vi "子VI-读取缺陷测量长宽和面积.vi"(10 "Particle Reports (Pixels)":T1(array[cluster]) {"Orientation" format="%.2f"; "Dimensions"."Height" format="%.2f"; "Dimensions"."Width" format="%.2f"; "Center of Mass"."Y" format="%.2f"; "Center of Mass"."X" format="%.2f"; "Bounding Rect"."Bottom" format="%.2f"; "Bounding Rect"."Right" format="%.2f"; "Bounding Rect"."Top" format="%.2f"; "Bounding Rect"."Left" format="%.2f"; "Number of Holes" format="%.2f"; "Area" format="%.2f"}) -> (2 "测量结果":dbl[][](array[numeric]))   [LabVIEW 2018]
panel:
  out "补几列空数字":dbl[](array[numeric])
  out "高":dbl[](array[numeric])
  out "宽":dbl[](array[numeric])
  out "面积":dbl[](array[numeric])
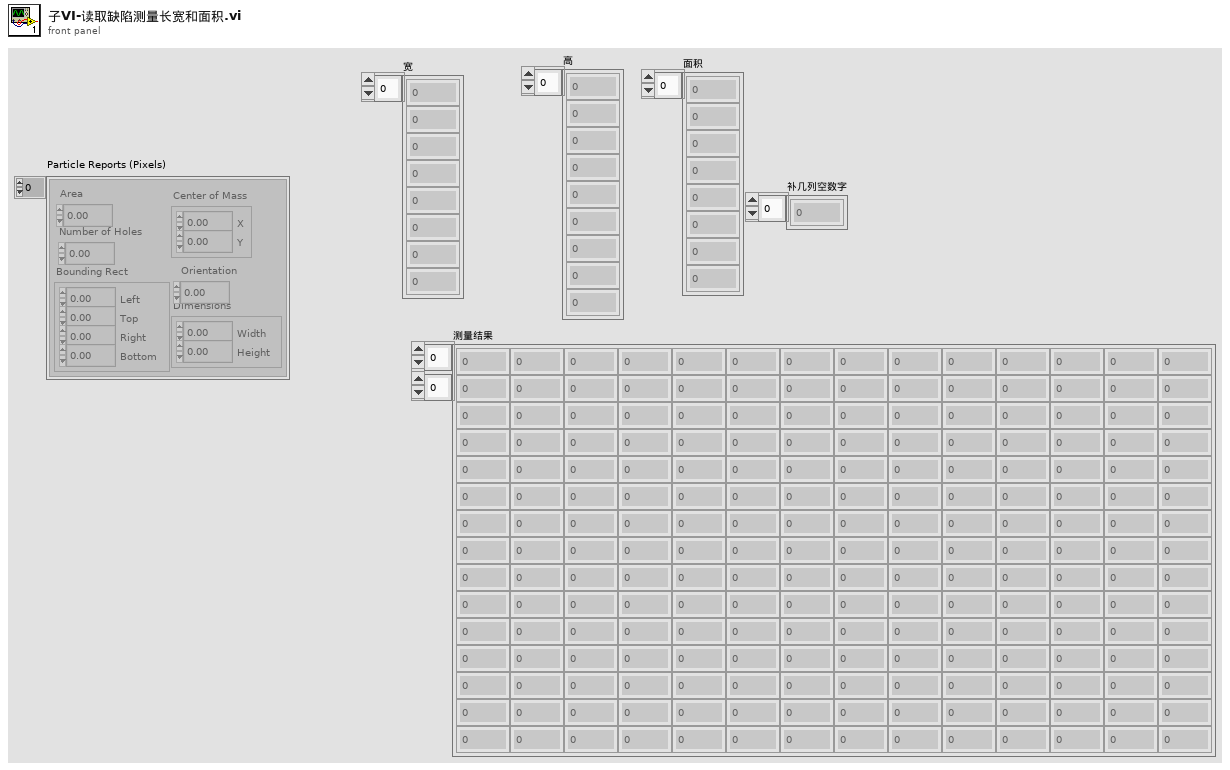
[diagram p1: front panel]
types:
  T1 = cluster{"Area":dbl, "Number of Holes":dbl, "Bounding Rect":cluster{"Left":dbl, "Top":dbl, "Right":dbl, "Bottom":dbl}, "Center of Mass":cluster{"X":dbl, "Y":dbl}, "Orientation":dbl, "Dimensions":cluster{"Width":dbl, "Height":dbl}}[]
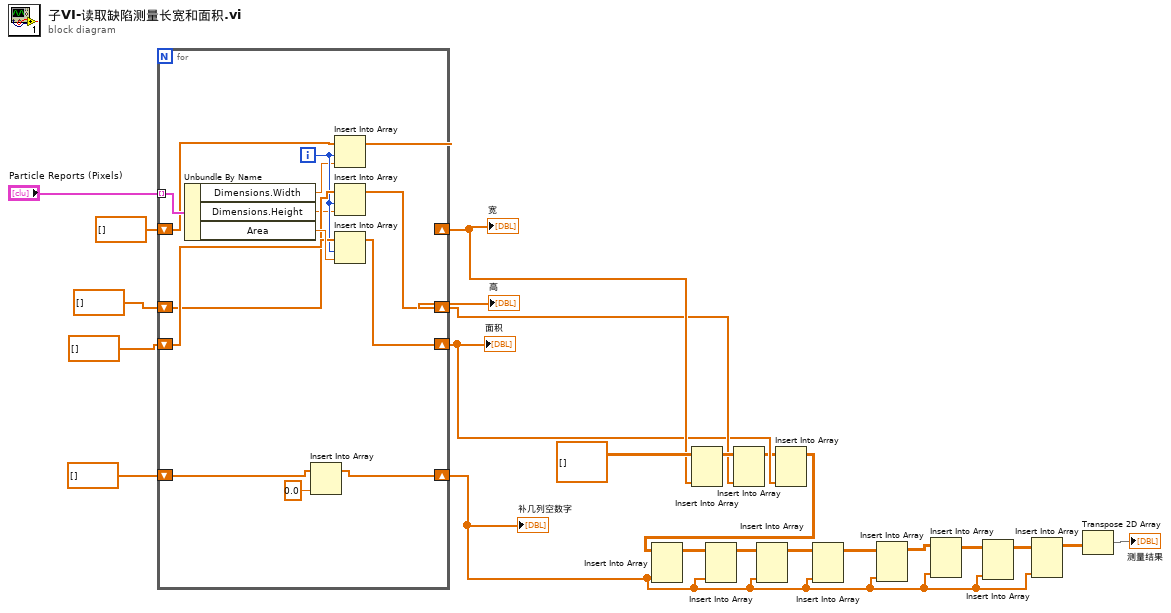
[diagram p0: block diagram]
diagram:
  n1 = for {
    tunnel: "Particle Reports (Pixels)" -> [w36] mode=indexing
    shift-right: [w33] -> w14
    shift-left: dbl[] [] ("数组") -> [w34]
    shift-right: [w28] -> w17
    shift-left: dbl[] [] ("数组") -> [w30]
    shift-right: [w29] -> w15
    shift-left: dbl[] [] ("数组") -> [w32]
    shift-right: [w23] -> w2
    shift-left: dbl[] [] ("数组") -> [w25]
    i -> [w31]
    n2 = Unbundle By Name(w36) -> ("Dimensions.Width"=w26:dbl, "Dimensions.Height"=w27:dbl, "Area"=w35:dbl)
    n3 = Insert Into Array(array=w25, new element=0.0 ("新元素/子数组")) -> (w23:dbl[])  [unwired: 1 in]
    n4 = Insert Into Array(array=w30, index=w31, new element=w26) -> (w28:dbl[])
    n5 = Insert Into Array(array=w32, index=w31, new element=w27) -> (w29:dbl[])
    n6 = Insert Into Array(array=w34, index=w31, new element=w35) -> (w33:dbl[])
  }
  "面积" <- w14
  "宽" <- w17
  "高" <- w15
  "补几列空数字" <- w2
  n7 = Insert Into Array(array=dbl[][] [] ("数组"), new element=w17) -> (w16:dbl[][])  [unwired: 2 in]
  n8 = Insert Into Array(array=w16, new element=w15) -> (w13:dbl[][])  [unwired: 2 in]
  n9 = Insert Into Array(array=w13, new element=w14) -> (w10:dbl[][])  [unwired: 2 in]
  n10 = Insert Into Array(array=w10, new element=w2) -> (w9:dbl[][])  [unwired: 2 in]
  n11 = Insert Into Array(array=w9, new element=w2) -> (w8:dbl[][])  [unwired: 2 in]
  n12 = Insert Into Array(array=w8, new element=w2) -> (w7:dbl[][])  [unwired: 2 in]
  n13 = Insert Into Array(array=w7, new element=w2) -> (w6:dbl[][])  [unwired: 2 in]
  n14 = Insert Into Array(array=w6, new element=w2) -> (w5:dbl[][])  [unwired: 2 in]
  n15 = Insert Into Array(array=w5, new element=w2) -> (w4:dbl[][])  [unwired: 2 in]
  n16 = Insert Into Array(array=w4, new element=w2) -> (w3:dbl[][])  [unwired: 2 in]
  n17 = Insert Into Array(array=w3, new element=w2) -> (w1:dbl[][])  [unwired: 2 in]
  n18 = Transpose 2D Array(2D array=w1) -> (transposed array=→"测量结果":dbl[][])
